vi "testAttribute.vi"(8 "Error In":errorcluster, 10 "attribute":T1 items=["NoAttribute"=0, "IncludeReference"=1, "Symmetric"=2, "Floating"=4, "Inverted"=8], 11 "QwtScaleEngine In":refnum<class "QwtScaleEngine.lvclass">) -> (0 "Error Out":errorcluster, 2 "Value":bool, 3 "QwtScaleEngine Out":refnum<class "QwtScaleEngine.lvclass">)   [LabVIEW 2014, in "QwtScaleEngine.lvclass"]
doc: "LabVIEW-specific documentation is not yet available. See <b>https://qwt.sourceforge.io/class_qwt_scale_engine.html#testAttribute</b>"
uses:
  QwtScaleEngine.lvclass
  Attribute.ctl
  LQ Core/LQIdentity/LQIdentity.lvclass/LQIdentity.ctl
  LQ Core/LQ Core.lvlib
  LQ Core/LQIdentity/LQIdentity.lvclass
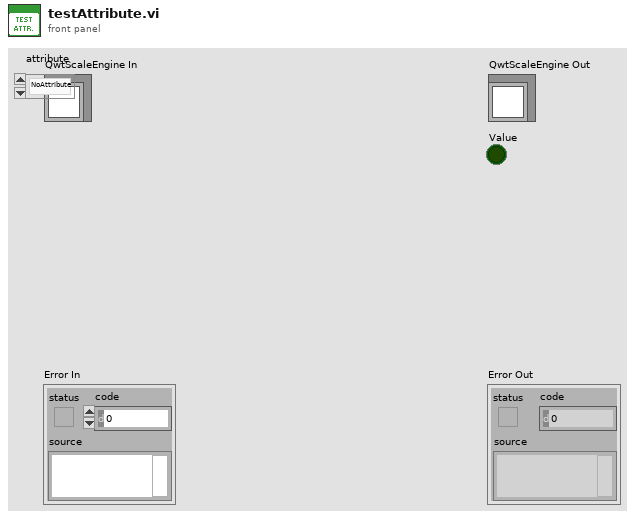
[diagram p1: front panel]
types:
  T1 = typedef "QwtScaleEngine.lvclass/Attribute.ctl" = i32
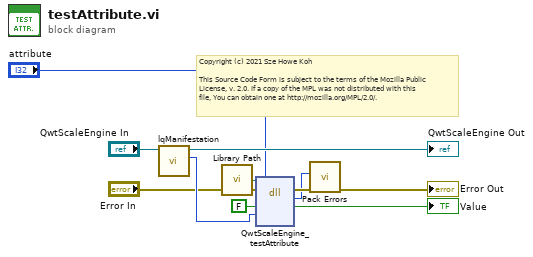
[diagram p0: block diagram]
diagram:
  # "Copyright (c) 2021 Sze Howe Koh\n\nThis Source Code Form is subject to the terms of the Mozilla Public\nLicense, v. 2.0. If a copy of the MPL was not distributed with this\nfile, You can obtain one at http://mozilla.org/MPL/2.0/."
  n1 = call "lqManifestation.vi"("LQIdentity in"="QwtScaleEngine In") -> ("Manifestation"=w6:u64, "LQIdentity out"=→"QwtScaleEngine Out":refnum<class "QwtScaleEngine.lvclass">)  [unwired: 9 in]
  n2 = call "Library Path.vi"() -> ("Library Path"=w7:path)
  n3 = dll-call lib="?" fn="QwtScaleEngine_testAttribute"(path in=w7, error in="Error In", "_retVal"=FALSE, "_instance"=w6, "attribute"="attribute") -> (error out=w4:errorcluster, w2:i32, "_retVal"=→"Value":bool)  [unwired: 3 in, 1 out]
  n4 = call "Pack Errors.vi"("Error In"=w4, "Error Code"=w2) -> ("Error Out"=→"Error Out":errorcluster)  [unwired: 9 in]
